vi "Webcam_GetImageData.vi"(8 "error in (no error)":errorcluster) -> (0 "error out":errorcluster, 2 "imagegray":u8[][](array[numeric]), 3 "image24bits":u32[][](array[numeric]))   [LabVIEW 2014, in "QwaveSys RPi Training Library.lvlib"]
uses:
  <vilib>/Q-Wave Systems/QwaveSys RPi Training Package (Demo)/Addons/QwaveSys RPi Training Library.lvlib
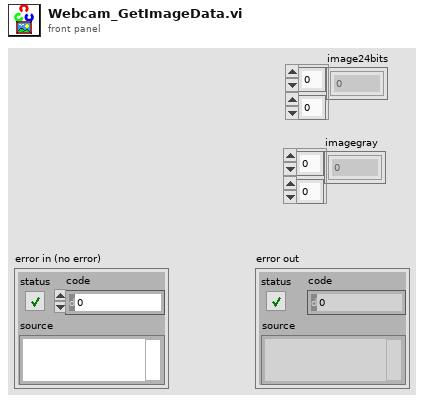
[diagram p1: front panel]
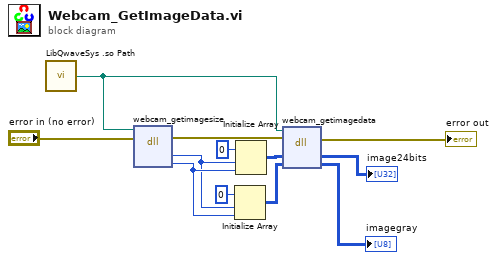
[diagram p0: block diagram]
diagram:
  n1 = call <vilib>:"LibQwaveSys .so Path.vi"() -> ("Lib QwaveSys .so Path"=w1:path)  [unwired: 5 in]
  n2 = dll-call lib="libqwavesys.so" fn="webcam_getimagesize"(path in=w1, error in="error in (no error)") -> (error out=w3:errorcluster, "rows"=w11:i32, "cols"=w12:i32)  [unwired: 4 in, 1 out]
  n3 = Initialize Array(u8 0 ("element"), w11, w12) -> (w10:u8[][])
  n4 = Initialize Array(u32 0 ("element"), w11, w12) -> (w8:u32[][])
  n5 = dll-call lib="libqwavesys.so" fn="webcam_getimagedata"(path in=w1, error in=w3, "image24bits"=w8, "imagegray"=w10) -> (error out=→"error out":errorcluster, "image24bits"=→"image24bits":u32[][], "imagegray"=→"imagegray":u8[][])  [unwired: 2 in, 1 out]
